vi "IsDeviceAccessible.vi"   [LabVIEW 2011, in "MvCameraControl.lvlib"]
uses:
  MvCameraControl.lvlib
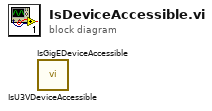
[diagram p0: block diagram]
diagram:
  n1 = call "IsU3VDeviceAccessible.vi"() -> ()  [unwired: 9 in, 2 out]
  n2 = call "IsGigEDeviceAccessible.vi"() -> ()  [unwired: 9 in, 2 out]
